vi "Image Fusion.vi"() -> ()   [LabVIEW 2023]
doc: "This example shows the application of the discrete wavelet transform (DWT) in image fusion.\n\nImage fusion merges images from different sources and modalities into a single image. The purpose of image fusion is to extract useful information from difference sources without introducing artifacts. The DWT-based image fusion method merges images in the wavelet-transform domain. The DWT method retains the sharp contrast information from all source images and provides both spatial and frequency localization. \n\nThis example computes the detail and approximation coefficients of two images with the WA Discrete Wavelet Transform VI, merges the resulting coefficients, and computes the fusion image with the WA Inverse Discrete Wavelet Transform VI.\n\n<b>Instructions:</b>\n1) Run this VI.\n2) Select a different <b>Fusion Method</b> and observe the <b>Fusion Image</b>."
uses:
  <vilib>/addons/Wavelet Analysis/typedefs.llb/WA Data.ctl
  <vilib>/addons/_Advanced Signal Processing/NI_AdvSigProcWA.lvlib
panel:
  in  "stop":bool
  out "Fusion Image":i32[][](graph)
  out "Image 2":u8[][](graph)
  out "Image 1":u8[][](graph)
  in  "Fusion method":cluster{"Approximation":u16, "Detail":u16} {"Detail" items=["Max", "Min", "Mean", "Image 1", "Image 2"]; "Approximation" items=["Max", "Min", "Mean", "Image 1", "Image 2"]}
  in  "Wavelet":u16(ring)=25 items=["Haar"=13, "bior2_2"=16, "bior4_4 (FBI)"=25]
  in  "Levels":i32=4
  # "Overview: Shows the application of the discrete wavelet transform (DWT) in image fusion.\nRequirements: LabVIEW Full Development System, Advanced Signal Processing Toolkit\nInstructions: \n1. Run this VI.\n2. Select a different Fusion Method and observe the Fusion Image.\n3. Click Stop to stop the VI."
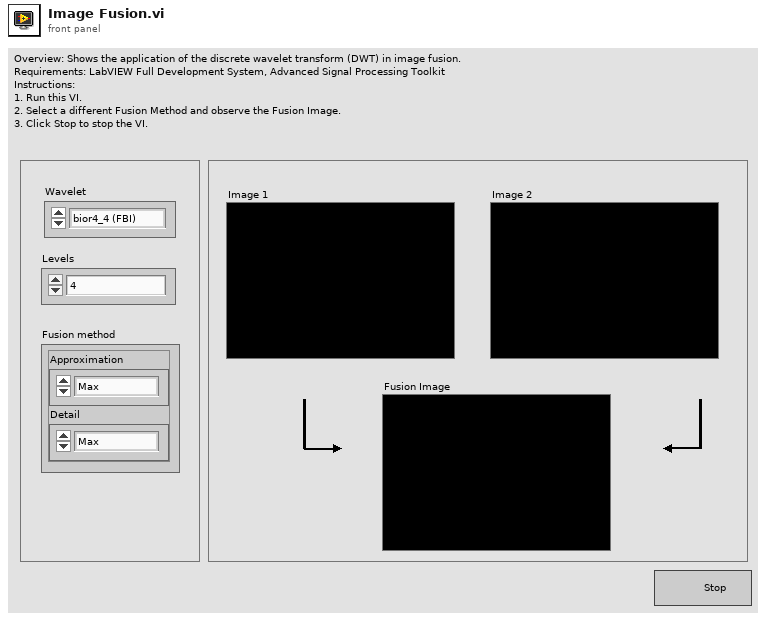
[diagram p1: front panel]
types:
  T1 = typedef "NI_AdvSigProcWA.lvlib/WA Data.ctl" = u16
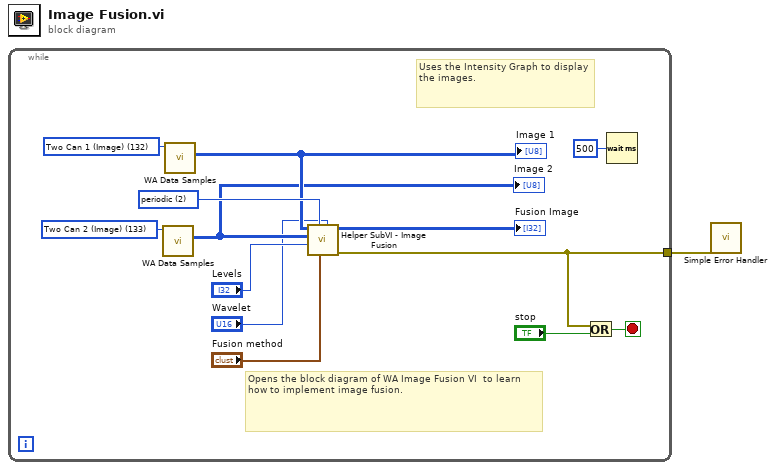
[diagram p0: block diagram]
diagram:
  n1 = while {
    tunnel: [w3] -> w1
    stop <- w9 stop-if-true
    w4 = T1 133 items=["1D Example Data"=100, "-"=101, "Doppler"=102, "HOP"=103, "TF Sine"=104, "Noisy Doppler"=105, "Sea Temperature"=106, "Sp500"=107, "Power Line"=108, "Engine Knocking"=109, "HeaviSine"=110, "Bumps"=111, "Blocks"=112, "Piece Regular"=113, "HypChirps"=114, "LinChirps"=115, "Chirps"=116, "Piece Polynomial"=117, "ECG"=131, "-"=118, "2D Example Data"=119, "-"=120, "Finger Print (Image)"=121, "Iris Flower (Image)"=122, "Mammogram (Image)"=123, "Lake (Image)"=127, "Two Can 1 (Image)"=132, "Two Can 2 (Image)"=133, "Camera Man (Image)"=134] ("data")
    w5 = T1 132 items=["1D Example Data"=100, "-"=101, "Doppler"=102, "HOP"=103, "TF Sine"=104, "Noisy Doppler"=105, "Sea Temperature"=106, "Sp500"=107, "Power Line"=108, "Engine Knocking"=109, "HeaviSine"=110, "Bumps"=111, "Blocks"=112, "Piece Regular"=113, "HypChirps"=114, "LinChirps"=115, "Chirps"=116, "Piece Polynomial"=117, "ECG"=131, "-"=118, "2D Example Data"=119, "-"=120, "Finger Print (Image)"=121, "Iris Flower (Image)"=122, "Mammogram (Image)"=123, "Lake (Image)"=127, "Two Can 1 (Image)"=132, "Two Can 2 (Image)"=133, "Camera Man (Image)"=134] ("data")
    w14 = u16 2 items=["zero padding", "symmetric", "periodic"] ("extension")
    # "Uses the Intensity Graph to display the images."
    # "Opens the block diagram of WA Image Fusion VI  to learn how to implement image fusion."
    n2 = call <vilib>:"WA Data Samples.vi"("data"=w4) -> ("image"=w6:u8[][])  [unwired: 10 out]
    "Image 2" <- w6
    n3 = call <vilib>:"WA Data Samples.vi"("data"=w5) -> ("image"=w7:u8[][])  [unwired: 10 out]
    "Image 1" <- w7
    n4 = call "Helper SubVI - Image Fusion.vi"("wavelet"="Wavelet", "fusion method"="Fusion method", "extension"=w14, "level"="Levels", "Image 2"=w6, "Image 1"=w7) -> ("error out"=w3:errorcluster, "Fusion Image"=→"Fusion Image":i32[][])  [unwired: 1 in, 3 out]
    n5 = Or(x=w3, y="stop") -> (x .or. y?=w9:bool)
    n6 = Wait (ms)(milliseconds to wait=u32 500 ("millisecond multiple")) -> ()  [unwired: 1 out]
  }
  n7 = call <vilib>:"Simple Error Handler.vi"("error in (no error)"=w1) -> ()  [unwired: 1 in, 8 out]
